vi "task_scheduler_test.vi"() -> ()   [LabVIEW 2015]
uses:
  <vilib>/Instr/_visa.llb/Select Event Type.ctl
  <vilib>/Utility/NIReport.llb/NI_report.lvclass
  <instrlib>/Agilent N6700 Series/Agilent N6700 Series.lvlib
  utilities/Test_Code/Global 5.vi
  utilities/Test_Code/Serial - Settings.ctl
  utilities/Test_Code/Serial - ASCII Characters.ctl
  utilities/Test_Code/Serial - XON-XOFF Characters.ctl
panel:
  out "Boolean":bool
  in  "Eclipse Load Current (A)":dbl=-0.1
  out "Protection Register":dbl[](graph)
  out "Input Power":dbl[](graph)
  out "Battery Charge":dbl[](graph)
  out "Battery Current Waveform":dbl[](graph)
  out "Solar Panel Current Waveform":dbl[](graph)
  out "Solar Panel Voltage Waveform":dbl[](graph)
  out "Battery Voltage Waveform":dbl[](graph)
  out "LED Current Waveform":dbl[](graph)
  in  "Load Current Step(A)":dbl=0.01 format="%#_13g"
  in  "Max. Load Current(A)":dbl=-0.5 format="%#_13g"
  in  "Time in eclipse (s)":dbl=2122.0 format="%#_13g"
  in  "Start":bool
  out "Action":string
  out "Load Current Waveform":dbl[](graph)
  out "Hour":i32
  out "Minute":i32
  out "Second":i32
  out "Fractional Second":dbl format="%#.4g"
  out "Count":i32
  out "Current Measurement":dbl format="%^.3e"
  in  "Negative Voltage Limit (0.0 volts)":dbl format="%^.3e"
  in  "Priority (1: Voltage)":i32(ring) items=["Voltage"=1, "Current"=0]
  in  "Positive Voltage Limit  (5.0 V)":dbl=5.0 format="%^.3e"
  in  "Channel Name (1)":string="4"
  in  "VISA resource name":refnum<visa-resource-name>="USB0::0x0957::0x0F07::MY53002228::INSTR"
  in  "stop":bool
  in  "report file path":path=path "C:/Users/Tulio/Documents/Testes/Backup excel/backup excel.xlsx"
  out "read buffer":string
  in  "Read Count":u32=1000
  in  "Termination Character":u8=10 format="%.0x"
  in  "End Write on Termination Character?":bool=TRUE
  in  "VISA resource name 2":refnum<visa-resource-name>="COM27"
  in  "XON/XOFF Characters":T1={"XON"=enum."DC1", "XOFF"=enum."DC3"}
  in  "Serial Settings":T3={"baud rate"=9600, "data bits"=8, "parity"=enum."None", "stop bits"=10, "flow control"=0} {"flow control" items=["None"=0, "XON/XOFF"=1, "RTS/CTS"=2, "DTR/DSR"=4]; "stop bits" items=["1.0"=10, "1.5"=15, "2.0"=20]; "data bits" min=5 max=8 step=1; "baud rate" items=["75"=75, "110"=110, "134"=134, "150"=150, "300"=300, "600"=600, "1200"=1200, "1800"=1800, "2400"=2400, "4800"=4800, "7200"=7200, "9600"=9600, "14400"=14400, "19200"=19200, "28800"=28800, "38400"=38400, "56000"=56000, "57600"=57600, "115200"=115200, "128000"=128000, "230400"=230400]}
  in  "End Read on Termination Character?":bool=TRUE
  # "More Graphs\n   ------------>"
  # "Chanel 1 -> Cooler source\nChannel 2-> LED source\nChanel 3 -> Board 3V3 source \nChannel 4 -> Load"
  # "Simulation Parameters"
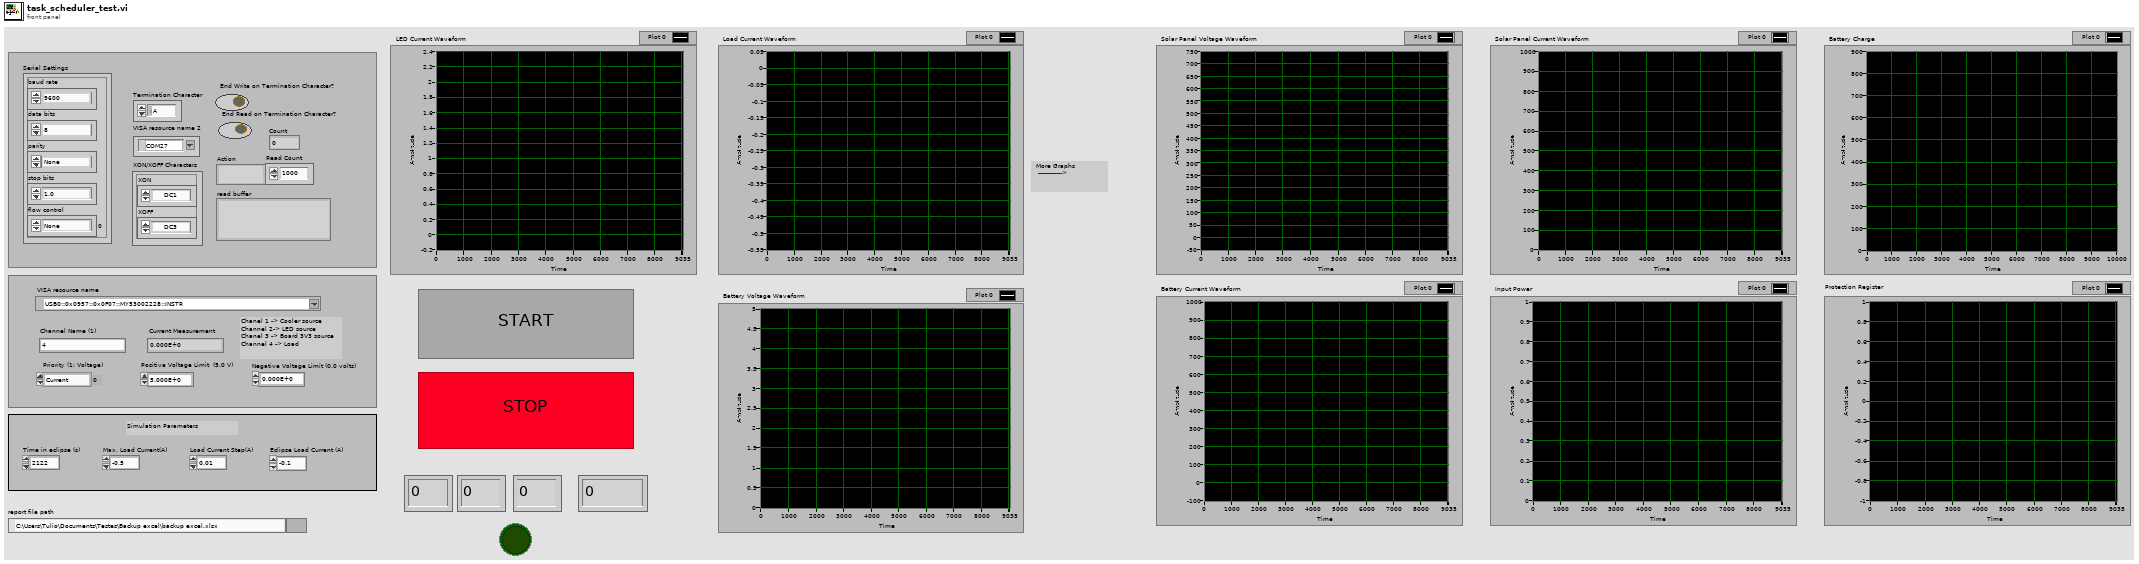
[diagram p1: front panel]
types:
  T1 = typedef "Serial - XON-XOFF Characters.ctl" = cluster{"XON":T2, "XOFF":T2}
  T2 = typedef "Serial - ASCII Characters.ctl" = enum16{"NUL", "SOH", "STX", "ETX", "EOT", "ENQ", "ACK", "BEL", "BS", "HT", "LF", "VT", "FF", "CR", "SO", "SI", "DLE", "DC1", "DC2", "DC3", "DC4", "NAK", "SYN", "ETB", "CAN", "EM", "SUB", "ESC", "FS", "GS", "RS", "US", "SP", "!", "\"", "#", "$", "%", "&", "'", "(", ")", "*", "+", ",", "- (-)", ".", "/", "0", "1", "2", "3", "4", "5", "6", "7", "8", "9", ":", ";", "<", "=", ">", "?", "@", "A", "B", "C", "D", "E", "F", "G", "H", "I", "J", "K", "L", "M", "N", "O", "P", "Q", "R", "S", "T", "U", "V", "W", "X", "Y", "Z", "[", "\\", "]", "^", "_", "`", "a", "b", "c", "d", "e", "f", "g", "h", "i", "j", "k", "l", "m", "n", "o", "p", "q", "r", "s", "t", "u", "v", "w", "x", "y", "z", "{", "|", "}", "~"}
  T3 = typedef "Serial - Settings.ctl" = cluster{"baud rate":u32, "data bits":u16, "parity":enum16{"None", "Odd", "Even", "Mark", "Space"}, "stop bits":u16, "flow control":u16}
  T4 = enum16{"Standard Report", "HTML", "Word", "Excel"}
  T5 = typedef "Select Event Type.ctl" = u32
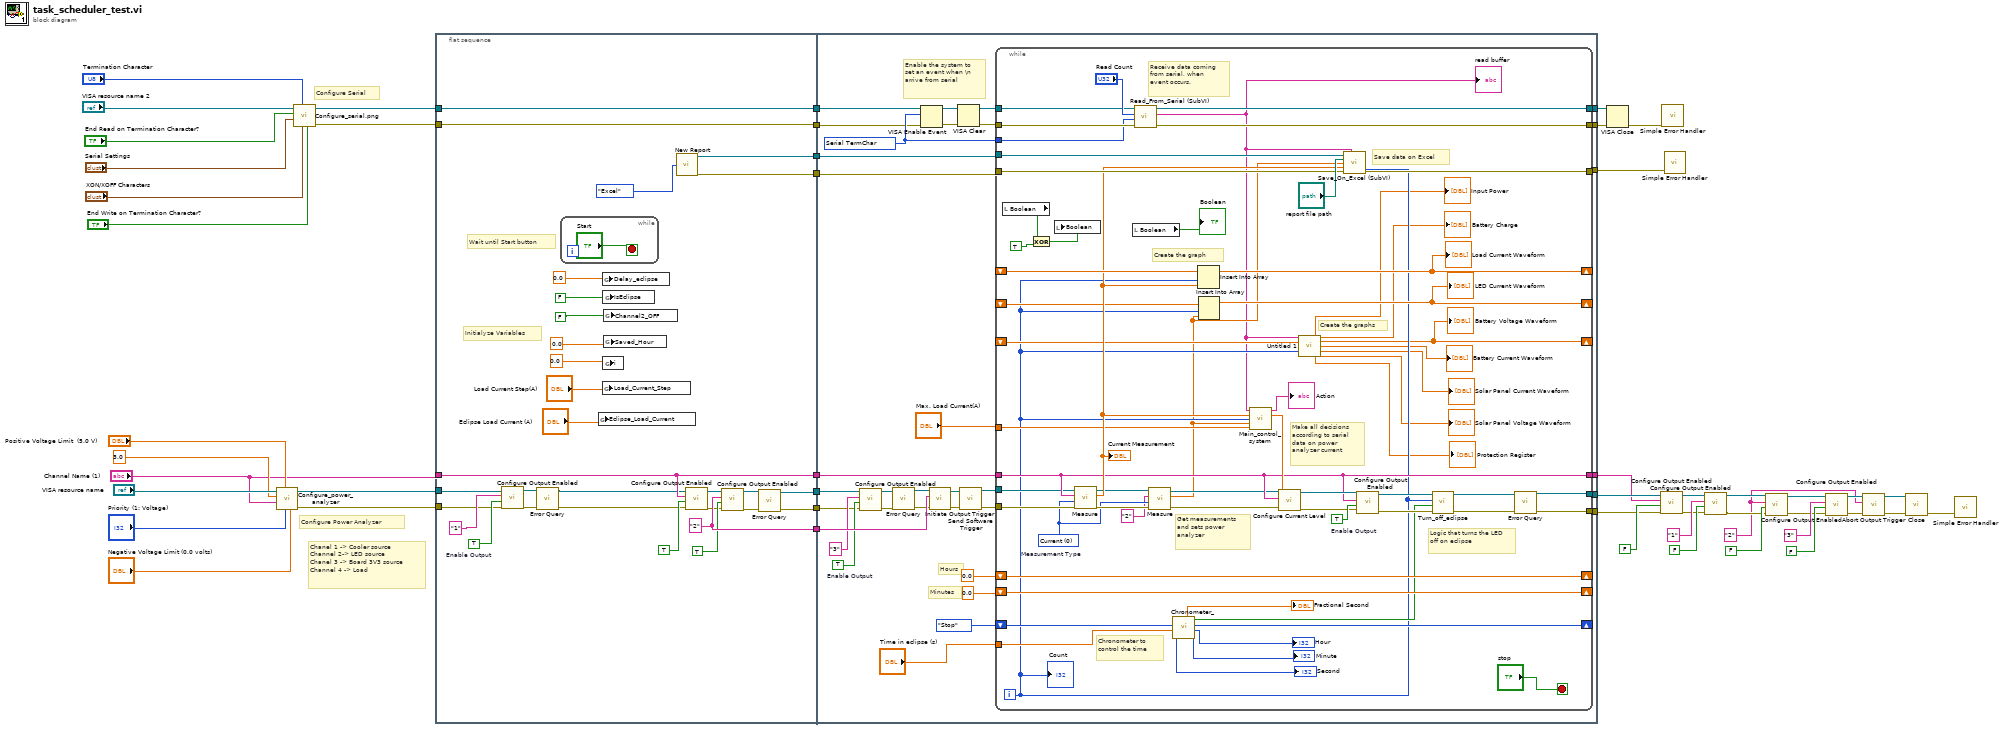
[diagram p0: block diagram]
diagram:
  w2 = "2" ("Channel Name (1)")
  # "Chanel 1 -> Cooler source\nChannel 2-> LED source\nChanel 3 -> Board 3V3 source \nChannel 4 -> Load"
  # "Configure Power Analyzer"
  # "Configure Serial"
  n1 = call "Configure_power_analyzer.vi"("Negative Voltage Limit (0.0 volts)"="Negative Voltage Limit (0.0 volts)", "Priority (1: Voltage)"="Priority (1: Voltage)", "Positive Voltage Limit  (5.0 V)"="Positive Voltage Limit  (5.0 V)", "Channel Name (1)"="Channel Name (1)", "Range (0.0)"=3.0, "VISA Refnum in"="VISA resource name") -> ("error out"=w8:errorcluster, "VISA Refnum out"=w9:refnum<visa-resource-name>)  [unwired: 4 in]
  n2 = call "Configure_serial.png"("End Write on Termination Character?"="End Write on Termination Character?", "XON/XOFF Characters"="XON/XOFF Characters", "Termination Character"="Termination Character", "Serial Settings"="Serial Settings", "End Read on Termination Character?"="End Read on Termination Character?", "VISA Refnum in"="VISA resource name 2") -> ("error out"=w12:errorcluster, "VISA Refnum out"=w13:refnum<visa-resource-name>)  [unwired: 4 in]
  n3 = flat-sequence {
    tunnel: "Channel Name (1)" -> [w65]
    tunnel: [w55] -> w18
    tunnel: [w56] -> w17
    tunnel: [w65] -> w16
    tunnel: [w79] -> w15
    tunnel: [w78] -> w14
    tunnel: w13 -> [w55]
    tunnel: w12 -> [w56]
    tunnel: [w58] -> w11
    tunnel: [w57] -> w10
    tunnel: w9 -> [w67]
    tunnel: w8 -> [w66]
    tunnel: [w63] -> w1
    tunnel: [w114] -> w44
    tunnel: [w113] -> w43
    tunnel: [w112] -> w40
    tunnel: [w108] -> w20
    tunnel: [w107] -> w19
    tunnel: w18 -> [w94]
    tunnel: w17 -> [w93]
    tunnel: w16 -> [w109]
    tunnel: w15 -> [w105]
    tunnel: w14 -> [w104]
    tunnel: w11 -> [w88]
    tunnel: w10 -> [w89]
    tunnel: [w103] -> w7
    tunnel: w1 -> [w95]
    frame #0 {
      w63 = "2" ("Channel Name (1)")
      w71 = TRUE  # Enable Output
      # "Wait until Start button"
      # "Initialyze Variables"
      n4 = call <instrlib>:"Configure Output Enabled.vi"("error in (no error)"=w66, "Enable Output (False)"=w71, "Channel Name (1)"="1", "VISA resource name"=w67) -> ("error out"=w72:errorcluster, "VISA resource name out"=w70:refnum<visa-resource-name>)  [unwired: 6 in]
      n5 = call <instrlib>:"Error Query.vi"("VISA resource name"=w70, "error in (no error)"=w72) -> ("VISA resource name out"=w51:refnum<visa-resource-name>, "error out"=w52:errorcluster)  [unwired: 10 in, 2 out]
      n6 = while {
        stop <- "Start" stop-if-true
      }
      n7 = global write "Global 5.vi" "Eclipse_Load_Current"("Eclipse Load Current (A)") -> ()
      n8 = global write "Global 5.vi" "Delay_eclipse"(0.0 ("Delay_eclipse")) -> ()
      n9 = global write "Global 5.vi" "Load_Current_Step"("Load Current Step(A)") -> ()
      n10 = global write "Global 5.vi" "IsEclipse"(FALSE ("Boolean")) -> ()
      n11 = global write "Global 5.vi" "i"(0.0 ("i")) -> ()
      n12 = global write "Global 5.vi" "Channel2_OFF"(FALSE ("Boolean")) -> ()
      n13 = global write "Global 5.vi" "Saved_Hour"(0.0 ("Numeric")) -> ()
      n14 = call <vilib>:"New Report.vi"("report type"=T4."Excel") -> ("report out"=w79:refnum<class "NI_report.lvclass">, "error out"=w78:errorcluster)  [unwired: 13 in]
      n15 = call <instrlib>:"Configure Output Enabled.vi"("error in (no error)"=w52, "Enable Output (False)"=TRUE, "Channel Name (1)"=w65, "VISA resource name"=w51) -> ("error out"=w61:errorcluster, "VISA resource name out"=w64:refnum<visa-resource-name>)  [unwired: 6 in]
      n16 = call <instrlib>:"Configure Output Enabled.vi"("error in (no error)"=w61, "Enable Output (False)"=TRUE, "Channel Name (1)"=w63, "VISA resource name"=w64) -> ("error out"=w59:errorcluster, "VISA resource name out"=w60:refnum<visa-resource-name>)  [unwired: 6 in]
      n17 = call <instrlib>:"Error Query.vi"("VISA resource name"=w60, "error in (no error)"=w59) -> ("VISA resource name out"=w58:refnum<visa-resource-name>, "error out"=w57:errorcluster)  [unwired: 10 in, 2 out]
    }
    frame #1 {
      w91 = TRUE  # Enable Output
      w98 = T5 1073684516 items=["Service Request"=1073684491, "Trigger"=3221168138, "Clear"=1073684493, "VXI Signal"=1073684512, "VXI/VME Interrupt"=3221168161, "VXI/VME Sysfail"=1073684509, "VXI/VME Sysreset"=1073684510, "GPIB CIC"=1073684498, "GPIB Talk"=1073684499, "GPIB Listen"=1073684500, "PXI Interrupt"=1073684514, "Serial Break"=1073684515, "Serial TermChar"=1073684516, "Serial CTS"=1073684521, "Serial DSR"=1073684522, "Serial DCD"=1073684524, "Serial RI"=1073684526, "Serial Character"=1073684533, "USB Interrupt"=1073684535, "All Enabled"=1073709055] ("Event Type")
      # "Enable the system to set an event when \\n arrive from serial"
      # "Minutes"
      # "Hours"
      n18 = call <instrlib>:"Configure Output Enabled.vi"("error in (no error)"=w89, "Enable Output (False)"=w91, "Channel Name (1)"="3", "VISA resource name"=w88) -> ("error out"=w92:errorcluster, "VISA resource name out"=w87:refnum<visa-resource-name>)  [unwired: 6 in]
      n19 = call <instrlib>:"Error Query.vi"("VISA resource name"=w87, "error in (no error)"=w92) -> ("VISA resource name out"=w86:refnum<visa-resource-name>, "error out"=w85:errorcluster)  [unwired: 10 in, 2 out]
      n20 = VISA Enable Event(8:w93, 10:w98, 11:w94) -> (0:w82:errorcluster, 3:w81:refnum<visa-resource-name>)  [unwired: 1 in]
      n21 = call <instrlib>:"Initiate Output Trigger.vi"("error in (no error)"=w85, "Channel Name (1)"=w95, "VISA resource name"=w86) -> ("error out"=w101:errorcluster, "VISA resource name out"=w102:refnum<visa-resource-name>)  [unwired: 7 in]
      n22 = VISA Clear(VISA resource name=w81, error in (no error)=w82) -> (VISA resource name out=w84:refnum<visa-resource-name>, error out=w83:errorcluster)
      n23 = call <instrlib>:"Send Software Trigger.vi"("error in (no error)"=w101, "VISA resource name"=w102) -> ("error out"=w99:errorcluster, "VISA resource name out"=w100:refnum<visa-resource-name>)  [unwired: 8 in]
      n24 = while {
        tunnel: w98 -> [w173]
        tunnel: w105 -> [w169]
        tunnel: w104 -> [w168]
        tunnel: [w167] -> w112
        shift-right: [w157] -> _
        shift-left: 0.0 -> [w157]
        shift-right: [w158] -> _
        shift-left: 0.0 -> [w158]
        tunnel: w100 -> [w140]
        tunnel: w99 -> [w156]
        shift-right: [w155] -> _
        shift-left: enum16{"Count", "Stop", "Reset"}."Stop" ("Action") -> [w154]
        tunnel: w109 -> [w141]
        tunnel: [w148] -> w108
        tunnel: [w147] -> w107
        tunnel: w84 -> [w175]
        tunnel: [w172] -> w114
        tunnel: w83 -> [w174]
        tunnel: [w171] -> w113
        shift-right: [w145] -> _
        shift-left: _ -> [w146]
        tunnel: [w141] -> w103
        tunnel: "Max. Load Current(A)" -> [w139]
        tunnel: "Time in eclipse (s)" -> [w138]
        shift-right: [w130] -> _
        shift-left: _ -> [w131]
        shift-right: [w127] -> _
        shift-left: _ -> [w129]
        i -> [w128]
        stop <- "stop" stop-if-true
        w133 = 0 items=["Voltage"=1, "Current"=0]  # Measurement Type
        w165 = TRUE  # Enable Output
        # "Create the graphs"
        # "Make all decisions according to serial data on power analyzer current"
        # "Create the graph"
        # "Logic that turns the LED off on eclipse"
        # "Chronometer to control the time"
        # "Get measurements and sets power analyzer"
        # "Save data on Excel"
        # "Receive data coming from serial, when event occurs."
        n25 = local read "Boolean"() -> (w118:bool)
        n26 = Exclusive Or(1:TRUE ("y"), 2:w118) -> (0:w119:bool)
        n27 = local write "Boolean"(w119) -> ()
        n28 = call <instrlib>:"Measure.vi"("error in (no error)"=w156, "Measurement Type (1: Voltage)"=w133, "Channel Name (1)"=w141, "VISA resource name"=w140) -> ("error out"=w136:errorcluster, "Measurement"=w144:dbl, "VISA resource name out"=w137:refnum<visa-resource-name>)  [unwired: 5 in]
        "Current Measurement" <- w144
        n29 = local read "Boolean"() -> (→"Boolean":bool)
        n30 = call "Read_From_Serial (SubVI).vi"("error in (no error)"=w174, "Event Type"=w173, "Read Count"="Read Count", "VISA Refnum in"=w175) -> ("error out"=w171:errorcluster, "read buffer"=w115:string, "VISA Refnum out"=w172:refnum<visa-resource-name>)  [unwired: 4 in]
        "read buffer" <- w115
        n31 = call <instrlib>:"Measure.vi"("error in (no error)"=w136, "Measurement Type (1: Voltage)"=w133, "Channel Name (1)"="2", "VISA resource name"=w137) -> ("error out"=w134:errorcluster, "Measurement"=w120:dbl, "VISA resource name out"=w135:refnum<visa-resource-name>)  [unwired: 5 in]
        n32 = call "Chronometer_.vi"("Time in eclipse (s)"=w138, "Action"=w154) -> ("Minute"=→"Minute":i32, "Hour"=→"Hour":i32, "Action out"=w155:enum16{"Count", "Stop", "Reset"}, "Boolean"=w153:bool, "Fractional Second"=→"Fractional Second":dbl, "Second"=→"Second":i32)  [unwired: 2 in]
        n33 = Insert Into Array(array=w146, index=w128, new element=w144) -> (w145:dbl[])
        "Load Current Waveform" <- w145
        n34 = Insert Into Array(array=w131, index=w128, new element=w120) -> (w130:dbl[])
        "LED Current Waveform" <- w130
        n35 = call "Main_control_system.vi"("read buffer"=w115, "Measurement in"=w144, "Numeric"=w128, "Measurement channel 2"=w120, "Max. Load Current"=w139) -> ("Action"=→"Action":string, "Measurement out"=w143:dbl)  [unwired: 9 in]
        n36 = call <instrlib>:"Configure Current Level.vi"("error in (no error)"=w134, "Level  (0.0 A)"=w143, "Channel Name (1)"=w141, "VISA resource name"=w135) -> ("error out"=w163:errorcluster, "VISA resource name out"=w164:refnum<visa-resource-name>)  [unwired: 6 in]
        n37 = call "Untitled 1.vi"("read buffer"=w115, "Array in"=w129, "Numeric"=w128) -> ("Input Power"=→"Input Power":dbl[], "Protection Register"=→"Protection Register":dbl[], "Battery Charge"=→"Battery Charge":dbl[], "Array out"=w127:dbl[], "Battery current"=→"Battery Current Waveform":dbl[], "Solar Panel current"=→"Solar Panel Current Waveform":dbl[], "Solar Panel voltage"=→"Solar Panel Voltage Waveform":dbl[])  [unwired: 10 in]
        "Battery Voltage Waveform" <- w127
        n38 = call "Save_On_Excel (SubVI).vi"("NI_report in"=w169, "read buffer"=w115, "report file path"="report file path", "LED Measurement"=w120, "Load Measurement"=w144, "error in (no error)"=w168, "Numeric"=w128) -> ("error out"=w167:errorcluster)  [unwired: 8 in]
        n39 = call <instrlib>:"Configure Output Enabled.vi"("error in (no error)"=w163, "Enable Output (False)"=w165, "Channel Name (1)"=w141, "VISA resource name"=w164) -> ("error out"=w161:errorcluster, "VISA resource name out"=w162:refnum<visa-resource-name>)  [unwired: 6 in]
        n40 = call "Turn_off_eclipse.vi"("error in (no error)"=w161, "Boolean"=w153, "Numeric"=w128, "VISA Refnum in"=w162) -> ("error out"=w159:errorcluster, "VISA Refnum out"=w160:refnum<visa-resource-name>)  [unwired: 6 in]
        n41 = call <instrlib>:"Error Query.vi"("VISA resource name"=w160, "error in (no error)"=w159) -> ("VISA resource name out"=w148:refnum<visa-resource-name>, "error out"=w147:errorcluster)  [unwired: 10 in, 2 out]
        "Count" <- w128
      }
    }
  }
  n42 = VISA Close(VISA resource name=w44, error in (no error)=w43) -> (error out=w45:errorcluster)
  n43 = call <instrlib>:"Configure Output Enabled.vi"("error in (no error)"=w19, "Enable Output (False)"=FALSE, "Channel Name (1)"=w7, "VISA resource name"=w20) -> ("error out"=w28:errorcluster, "VISA resource name out"=w27:refnum<visa-resource-name>)  [unwired: 6 in]
  n44 = call <vilib>:"Simple Error Handler.vi"("error in (no error)"=w45) -> ()  [unwired: 1 in, 8 out]
  n45 = call <vilib>:"Simple Error Handler.vi"("error in (no error)"=w40) -> ()  [unwired: 1 in, 8 out]
  n46 = call <instrlib>:"Configure Output Enabled.vi"("error in (no error)"=w28, "Enable Output (False)"=FALSE, "Channel Name (1)"="1", "VISA resource name"=w27) -> ("error out"=w30:errorcluster, "VISA resource name out"=w31:refnum<visa-resource-name>)  [unwired: 6 in]
  n47 = call <instrlib>:"Configure Output Enabled.vi"("error in (no error)"=w30, "Enable Output (False)"=FALSE, "Channel Name (1)"=w2, "VISA resource name"=w31) -> ("error out"=w23:errorcluster, "VISA resource name out"=w22:refnum<visa-resource-name>)  [unwired: 6 in]
  n48 = call <instrlib>:"Configure Output Enabled.vi"("error in (no error)"=w23, "Enable Output (False)"=FALSE, "Channel Name (1)"="3", "VISA resource name"=w22) -> ("error out"=w3:errorcluster, "VISA resource name out"=w4:refnum<visa-resource-name>)  [unwired: 6 in]
  n49 = call <instrlib>:"Abort Output Trigger.vi"("error in (no error)"=w3, "Channel Name (1)"=w2, "VISA resource name"=w4) -> ("error out"=w5:errorcluster, "VISA resource name out"=w6:refnum<visa-resource-name>)  [unwired: 7 in]
  n50 = call <instrlib>:"Close.vi"("VISA resource name"=w6, "error in (no error)"=w5) -> ("error out"=w26:errorcluster)  [unwired: 13 in]
  n51 = call <vilib>:"Simple Error Handler.vi"("error in (no error)"=w26) -> ()  [unwired: 4 in, 5 out]
